vi "Data Convert.vi"(8 "error in (no error)":errorcluster, 11 "Array 2":string[][](array[string])=[["0.00056", "0.00066", "-0.00083", "-0.00131", "0.00150", "0.00018", "0.00022", "-0.00010", "-0.10252", "0.00033", "-0.00037", "-1.41487", "0.00019", "1.27792", "0.00062", "0.00263"], ["-0.00079", "-0.00021", "-0.00155", "-0.00166", "0.00078", "-0.00007", "0.00007", "-0.00024", "-0.10592", "0.00045", "0.00043", "-1.38900", "0.00024", "1.27712", "0.00062", "-0.00370"], ["0.09143", "0.10973", "0.12193", "0.11707", "0.10433", "0.10976", "0.12103", "-0.00023", "0.00443", "0.09399", "0.10549", "-1.38377", "0.00060", "1.38264", "0.08182", "0.10352"], ["-0.00028", "0.00087", "-0.00111", "-0.00220", "0.00094", "0.00053", "0.00031", "-0.00002", "-0.11705", "0.00019", "-0.00057", "-1.41933", "0.00021", "1.27317", "0.00104", "0.00493"], ["0.19056", "0.19841", "0.23113", "0.22792", "0.23177", "0.15519", "0.20205", "-0.00018", "0.10206", "0.17896", "0.20447", "-1.38386", "-0.00001", "1.37202", "0.18677", "0.20474"], ["-0.00042", "0.00070", "-0.00132", "-0.00189", "0.00038", "0.00049", "0.00077", "-0.00022", "-0.11917", "-0.00010", "-0.00010", "-1.42027", "0.00023", "1.26914", "0.00067", "-0.00174"], ["0.37911", "0.45323", "0.45892", "0.43110", "0.41458", "0.40783", "0.42956", "-0.00013", "0.26828", "0.43993", "0.32999", "-1.38627", "0.00018", "1.38414", "0.36010", "0.40861"], ["-0.00045", "0.00058", "-0.00138", "-0.00175", "0.00041", "0.00032", "0.00014", "0.00003", "-0.12137", "0.00033", "0.00026", "-1.38799", "0.00020", "1.26699", "0.00107", "0.00072"], ["0.76390", "0.87558", "0.76343", "0.80423", "0.86065", "0.80312", "0.89825", "0.00011", "0.70528", "0.88428", "0.70936", "-1.41689", "0.00043", "2.10535", "0.79408", "0.77772"], ["0.00013", "0.00049", "-0.00149", "-0.00192", "0.00069", "0.00033", "0.00047", "-0.00001", "-0.12205", "0.00060", "0.00043", "-1.42059", "-0.00014", "1.26665", "0.00136", "-0.00061"], ["0.76689", "0.86743", "0.94002", "0.79688", "0.90823", "0.79625", "0.70321", "0.00002", "0.67990", "0.82658", "0.76131", "-1.38877", "0.00029", "1.24913", "0.70545", "0.90097"], ["0.00024", "0.00025", "-0.00126", "-0.00202", "0.00085", "0.00019", "0.00051", "-0.00015", "-0.12322", "0.00005", "0.00000", "-1.38455", "0.00025", "1.25022", "-0.00018", "0.00176"], ["0.77855", "0.87510", "0.85246", "0.85461", "0.86674", "0.75010", "0.88420", "0.00020", "0.43106", "0.86739", "0.80059", "-1.38297", "0.00029", "1.35980", "0.76460", "0.83495"], ["-0.00053", "0.00103", "-0.00129", "-0.00239", "0.00093", "0.00065", "0.00072", "0.00009", "-0.13199", "0.00025", "-0.00011", "-1.41408", "-0.00004", "1.25102", "0.00070", "0.00035"], ["0.78238", "0.85177", "0.71040", "0.75267", "0.66687", "0.74783", "0.93722", "-0.00001", "0.61890", "0.90562", "0.75812", "-1.41743", "0.00006", "1.76053", "0.74920", "0.90033"], ["-0.00027", "0.00106", "-0.00123", "-0.00164", "0.00130", "-0.00010", "0.00098", "0.00034", "-0.13332", "0.00061", "-0.00019", "-1.42007", "0.00010", "1.24214", "0.00051", "0.00139"], ["0.18979", "0.19828", "0.18824", "0.16663", "0.20885", "0.19999", "0.23266", "-0.00033", "0.05098", "0.21080", "0.18429", "-1.38920", "0.00023", "1.44943", "0.17756", "0.24196"], ["0.00085", "0.00070", "-0.00140", "-0.00192", "0.00036", "0.00006", "0.00080", "0.00009", "-0.13420", "0.00039", "0.00020", "-1.38747", "-0.00010", "1.24261", "0.00074", "0.00357"], ["0.19763", "0.22276", "0.20829", "0.25512", "0.23264", "0.15552", "0.24704", "0.00015", "0.07936", "0.20765", "0.21202", "-1.41750", "-0.00002", "1.43976", "0.17056", "0.23740"], ["-0.00038", "0.00117", "-0.00119", "-0.00215", "0.00085", "0.00038", "0.00040", "0.00001", "-0.13548", "0.00014", "0.00036", "-1.38784", "0.00013", "1.24143", "0.00116", "0.00707"], ["0.36845", "0.43586", "0.45516", "0.35518", "0.36958", "0.35969", "0.38596", "-0.00010", "0.29444", "0.46509", "0.36984", "-1.41514", "0.00031", "1.61803", "0.38886", "0.35426"], ["-0.00008", "0.00024", "-0.00154", "-0.00186", "0.00093", "0.00015", "0.00048", "-0.00002", "-0.13660", "-0.00007", "0.00014", "-1.41942", "0.00058", "1.25677", "0.00096", "-0.00403"], ["0.75510", "0.81608", "0.91526", "0.84361", "0.91151", "0.76652", "0.75509", "0.00002", "0.72431", "0.90224", "0.74364", "-1.38721", "0.00045", "1.97083", "0.79778", "0.78490"], ["-0.00039", "0.00100", "-0.00137", "-0.00228", "0.00112", "0.00042", "0.00057", "-0.00009", "-0.13741", "-0.00025", "0.00005", "-1.38289", "0.00004", "1.26163", "0.00042", "0.00581"], ["0.71421", "0.79671", "0.90219", "0.83159", "0.89456", "0.73737", "0.89563", "0.00037", "0.68989", "0.79356", "0.71602", "-1.41746", "-0.00006", "2.05963", "0.74262", "0.86651"], ["0.00050", "-0.00011", "-0.00097", "-0.00179", "0.00098", "0.00021", "0.00012", "0.00018", "-0.13786", "0.00034", "-0.00023", "-1.41778", "0.00019", "1.27797", "0.00035", "0.00033"], ["3.75085", "4.22431", "4.08030", "3.99107", "4.04531", "3.76195", "4.16826", "0.00000", "3.52780", "4.19238", "3.66500", "-1.38738", "0.00042", "2.90096", "3.63501", "4.11336"], ["-0.00047", "0.00040", "-0.00117", "-0.00080", "0.00115", "0.00014", "0.00100", "-0.00004", "-0.13555", "0.00046", "0.00050", "-1.38689", "0.00029", "1.21243", "0.00063", "0.00603"], ["2.22423", "2.46898", "2.66954", "2.45772", "2.61462", "2.21687", "2.51106", "-0.00008", "2.38022", "2.57703", "2.22290", "-1.41946", "0.00038", "3.49164", "2.27467", "2.46864"], ["-0.00009", "-0.00002", "-0.00075", "-0.00120", "0.00150", "0.00029", "0.00076", "-0.00025", "-0.13491", "0.00076", "0.00019", "-1.38477", "0.00060", "1.21630", "0.00122", "0.00356"]]) -> (0 "error out":errorcluster, 3 "Data Out":string[][](array[string]))   [LabVIEW 2012]
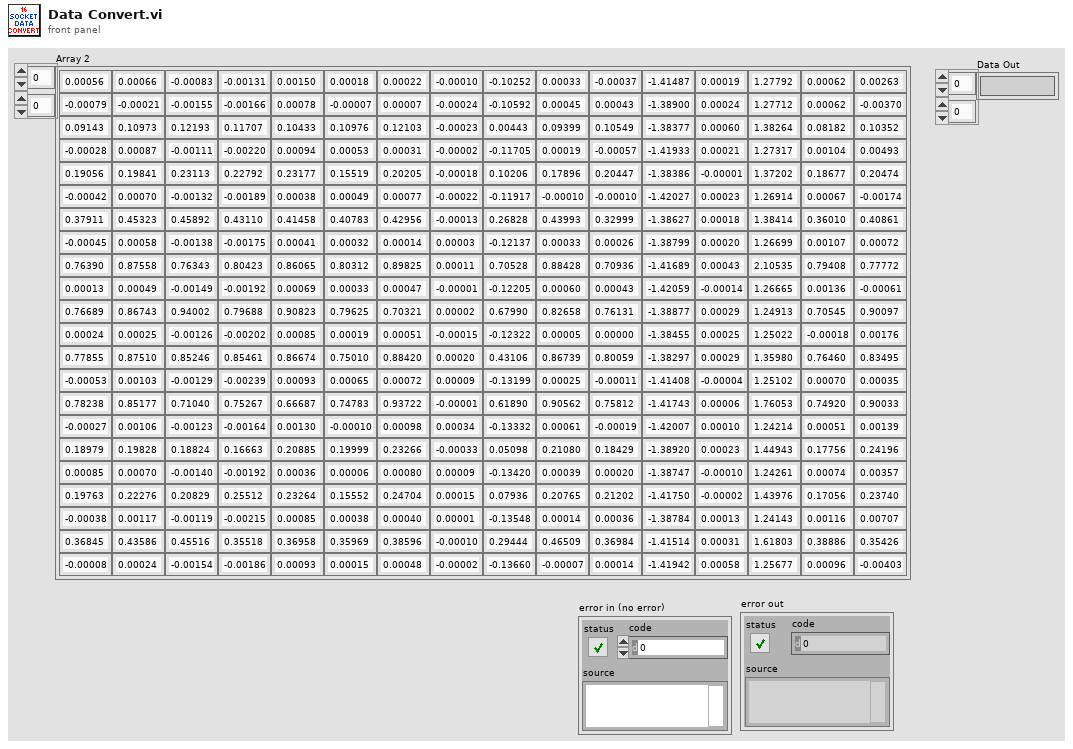
[diagram p1: front panel]
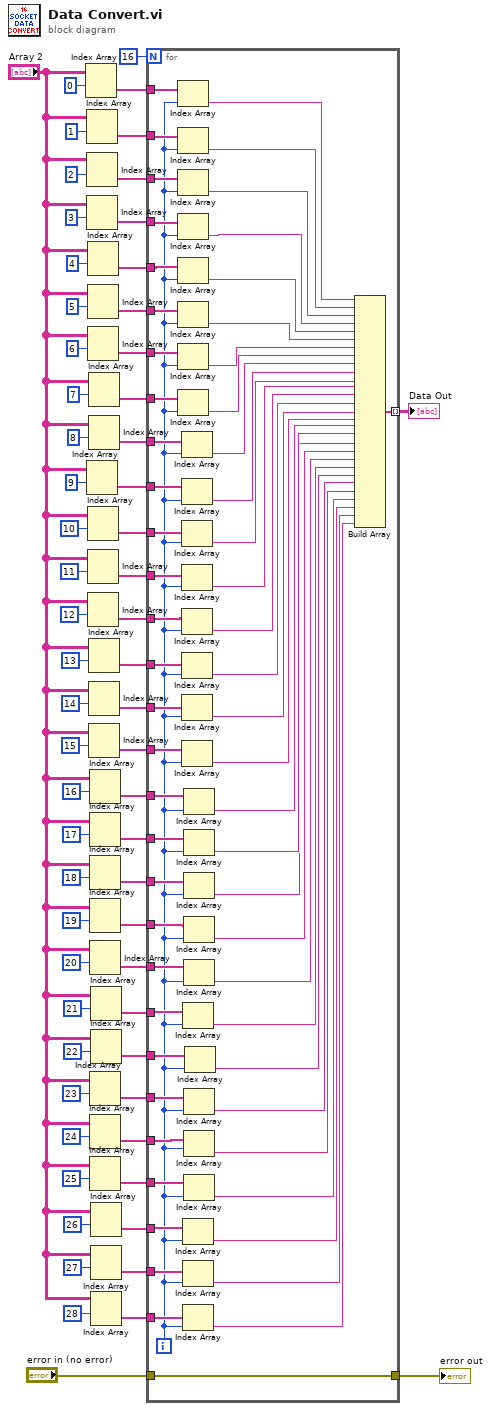
[diagram p0: block diagram]
diagram:
  n1 = Index Array(array="Array 2", index (row)=0) -> (element=w45:string[])  [unwired: 1 in]
  n2 = Index Array(array="Array 2", index (row)=1) -> (element=w44:string[])  [unwired: 1 in]
  n3 = Index Array(array="Array 2", index (row)=2) -> (element=w43:string[])  [unwired: 1 in]
  n4 = Index Array(array="Array 2", index (row)=3) -> (element=w42:string[])  [unwired: 1 in]
  n5 = Index Array(array="Array 2", index (row)=9) -> (element=w36:string[])  [unwired: 1 in]
  n6 = Index Array(array="Array 2", index (row)=4) -> (element=w41:string[])  [unwired: 1 in]
  n7 = Index Array(array="Array 2", index (row)=5) -> (element=w40:string[])  [unwired: 1 in]
  n8 = Index Array(array="Array 2", index (row)=6) -> (element=w39:string[])  [unwired: 1 in]
  n9 = Index Array(array="Array 2", index (row)=10) -> (element=w35:string[])  [unwired: 1 in]
  n10 = Index Array(array="Array 2", index (row)=11) -> (element=w34:string[])  [unwired: 1 in]
  n11 = Index Array(array="Array 2", index (row)=12) -> (element=w33:string[])  [unwired: 1 in]
  n12 = Index Array(array="Array 2", index (row)=7) -> (element=w38:string[])  [unwired: 1 in]
  n13 = Index Array(array="Array 2", index (row)=8) -> (element=w37:string[])  [unwired: 1 in]
  n14 = Index Array(array="Array 2", index (row)=13) -> (element=w32:string[])  [unwired: 1 in]
  n15 = Index Array(array="Array 2", index (row)=14) -> (element=w31:string[])  [unwired: 1 in]
  n16 = Index Array(array="Array 2", index (row)=15) -> (element=w30:string[])  [unwired: 1 in]
  n17 = Index Array(array="Array 2", index (row)=16) -> (element=w29:string[])  [unwired: 1 in]
  n18 = Index Array(array="Array 2", index (row)=17) -> (element=w28:string[])  [unwired: 1 in]
  n19 = Index Array(array="Array 2", index (row)=18) -> (element=w15:string[])  [unwired: 1 in]
  n20 = Index Array(array="Array 2", index (row)=19) -> (element=w14:string[])  [unwired: 1 in]
  n21 = Index Array(array="Array 2", index (row)=20) -> (element=w13:string[])  [unwired: 1 in]
  n22 = Index Array(array="Array 2", index (row)=23) -> (element=w10:string[])  [unwired: 1 in]
  n23 = Index Array(array="Array 2", index (row)=24) -> (element=w9:string[])  [unwired: 1 in]
  n24 = Index Array(array="Array 2", index (row)=25) -> (element=w8:string[])  [unwired: 1 in]
  n25 = Index Array(array="Array 2", index (row)=21) -> (element=w12:string[])  [unwired: 1 in]
  n26 = Index Array(array="Array 2", index (row)=22) -> (element=w11:string[])  [unwired: 1 in]
  n27 = Index Array(array="Array 2", index (row)=26) -> (element=w7:string[])  [unwired: 1 in]
  n28 = Index Array(array="Array 2", index (row)=27) -> (element=w6:string[])  [unwired: 1 in]
  n29 = Index Array(array="Array 2", index (row)=28) -> (element=w5:string[])  [unwired: 1 in]
  n30 = for {
    N: 16 -> [_]
    tunnel: w45 -> [w124]
    tunnel: w44 -> [w123]
    tunnel: w43 -> [w122]
    tunnel: w42 -> [w121]
    tunnel: w41 -> [w120]
    tunnel: w40 -> [w119]
    tunnel: w39 -> [w118]
    tunnel: w38 -> [w117]
    tunnel: w37 -> [w116]
    tunnel: w36 -> [w115]
    tunnel: w35 -> [w114]
    tunnel: w34 -> [w113]
    tunnel: w33 -> [w112]
    tunnel: w32 -> [w111]
    tunnel: w31 -> [w110]
    tunnel: w30 -> [w109]
    tunnel: w29 -> [w99]
    tunnel: w28 -> [w100]
    tunnel: w15 -> [w101]
    tunnel: w14 -> [w102]
    tunnel: w13 -> [w103]
    tunnel: w12 -> [w108]
    tunnel: w11 -> [w107]
    tunnel: w10 -> [w106]
    tunnel: w9 -> [w105]
    tunnel: w8 -> [w104]
    tunnel: w7 -> [w98]
    tunnel: w6 -> [w97]
    tunnel: w5 -> [w96]
    tunnel: [w65] -> w4 mode=indexing
    tunnel: [w64] -> w1
    tunnel: "error in (no error)" -> [w64]
    i -> [w95]
    n31 = Index Array(array=w124, index=w95) -> (element=w94:string)
    n32 = Index Array(array=w123, index=w95) -> (element=w93:string)
    n33 = Index Array(array=w122, index=w95) -> (element=w92:string)
    n34 = Index Array(array=w121, index=w95) -> (element=w91:string)
    n35 = Index Array(array=w120, index=w95) -> (element=w90:string)
    n36 = Index Array(array=w119, index=w95) -> (element=w89:string)
    n37 = Index Array(array=w118, index=w95) -> (element=w88:string)
    n38 = Index Array(array=w117, index=w95) -> (element=w87:string)
    n39 = Index Array(array=w116, index=w95) -> (element=w86:string)
    n40 = Index Array(array=w115, index=w95) -> (element=w85:string)
    n41 = Index Array(array=w114, index=w95) -> (element=w84:string)
    n42 = Index Array(array=w113, index=w95) -> (element=w83:string)
    n43 = Index Array(array=w112, index=w95) -> (element=w82:string)
    n44 = Index Array(array=w111, index=w95) -> (element=w81:string)
    n45 = Index Array(array=w110, index=w95) -> (element=w80:string)
    n46 = Index Array(array=w109, index=w95) -> (element=w79:string)
    n47 = Index Array(array=w108, index=w95) -> (element=w73:string)
    n48 = Index Array(array=w98, index=w95) -> (element=w68:string)
    n49 = Index Array(array=w97, index=w95) -> (element=w67:string)
    n50 = Index Array(array=w96, index=w95) -> (element=w66:string)
    n51 = Index Array(array=w99, index=w95) -> (element=w78:string)
    n52 = Index Array(array=w100, index=w95) -> (element=w77:string)
    n53 = Index Array(array=w101, index=w95) -> (element=w76:string)
    n54 = Index Array(array=w102, index=w95) -> (element=w75:string)
    n55 = Index Array(array=w103, index=w95) -> (element=w74:string)
    n56 = Index Array(array=w106, index=w95) -> (element=w71:string)
    n57 = Index Array(array=w105, index=w95) -> (element=w70:string)
    n58 = Index Array(array=w104, index=w95) -> (element=w69:string)
    n59 = Index Array(array=w107, index=w95) -> (element=w72:string)
    n60 = Build Array(w94, w93, w92, w91, w90, w89, w88, w87, w86, w85, w84, w83, w82, w81, w80, w79, w78, w77, w76, w75, w74, w73, w72, w71, w70, w69, w68, w67, w66) -> (w65:string[])
  }
  "Data Out" <- w4
  "error out" <- w1
